vi "Finish.vi"(8 "error in (no error)":errorcluster, 11 "Shooter One Wheel in":refnum<class "Shooter One Wheel.lvclass">) -> (0 "error out":errorcluster, 3 "Shooter One Wheel out":refnum<class "Shooter One Wheel.lvclass">)   [LabVIEW 2019, in "Shooter.lvlib" / "Shooter One Wheel.lvclass"]
uses:
  Shooter One Wheel.lvclass
  Shooter.lvclass
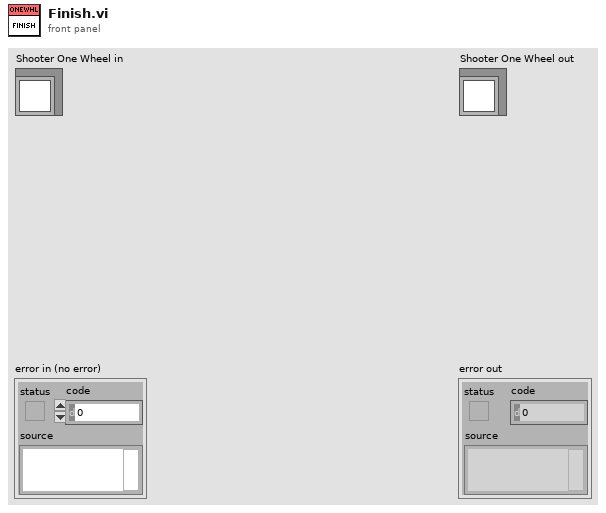
[diagram p1: front panel]
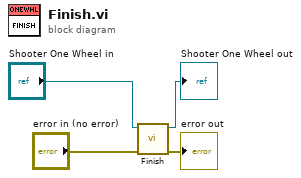
[diagram p0: block diagram]
diagram:
  n1 = call-parent "Finish.vi"("error in (no error)"="error in (no error)", "Shooter in"="Shooter One Wheel in") -> ("error out"=→"error out":errorcluster, "Shooter out"=→"Shooter One Wheel out":refnum<class "Shooter One Wheel.lvclass">)  [unwired: 8 in]
